vi "RichToFlatni_measurementlink_pinmap_v1_UpdatePinMapFromXmlRequest.vi"(5 "OutputClusterType":T1, 11 "InputCluster":T2) -> (3 "OutputCluster":T1)   [LabVIEW 2020, in "MeasurementLink Pin Map Client.lvlib"]
uses:
  MeasurementLink Pin Map Client.lvlib
  ni_measurementlink_pinmap_v1_UpdatePinMapFromXmlRequest.ctl
  ni_measurementlink_pinmap_v1_UpdatePinMapFromXmlRequest_Flat.ctl
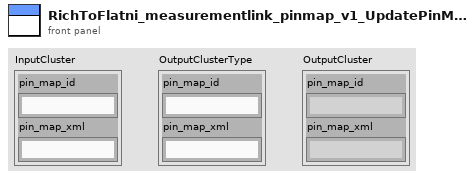
[diagram p1: front panel]
types:
  T1 = typedef "MeasurementLink Pin Map Client.lvlib/ni_measurementlink_pinmap_v1_UpdatePinMapFromXmlRequest_Flat.ctl" = cluster{"pin_map_id":string, "pin_map_xml":string}
  T2 = typedef "MeasurementLink Pin Map Client.lvlib/ni_measurementlink_pinmap_v1_UpdatePinMapFromXmlRequest.ctl" = cluster{"pin_map_id":string, "pin_map_xml":string}
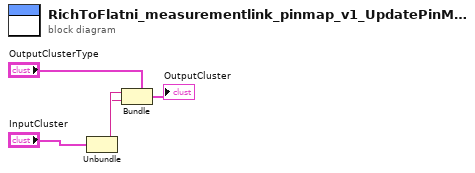
[diagram p0: block diagram]
diagram:
  n1 = Unbundle "Unbundle"("InputCluster") -> ("pin_map_id"=w2:string, "pin_map_xml"=w1:string)
  n2 = Bundle "Bundle"(cluster="OutputClusterType", "pin_map_id"=w2, "pin_map_xml"=w1) -> (→"OutputCluster":T1)
